vi "Untitled 1.vi"(0 "Cluster":cluster{"String":string}, 7 "Boolean":bool) -> ()   [LabVIEW 2015]
doc: "eedfgs"
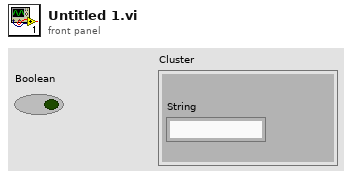
[diagram p1: front panel]
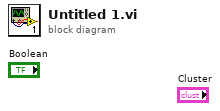
[diagram p0: block diagram]
diagram:
